vi "Error File Logger.vi"(0 "errlog Name":string="Errors.log", 1 "Module":string, 2 "Clear Error?":bool=TRUE, 3 "ContainerFolder(Empty for Application Folder)":path, 5 "error in (no error)":errorcluster) -> (4 "Error Log":string, 6 "error out":errorcluster)   [LabVIEW 2017]
doc: "Appends the error on the error in cluster to a log file, creating the folder and file when they do not exist, and returns the log text. Wire Clear Error? to clear the error after logging, and ContainerFolder to choose where the log is written (empty uses the application folder)."
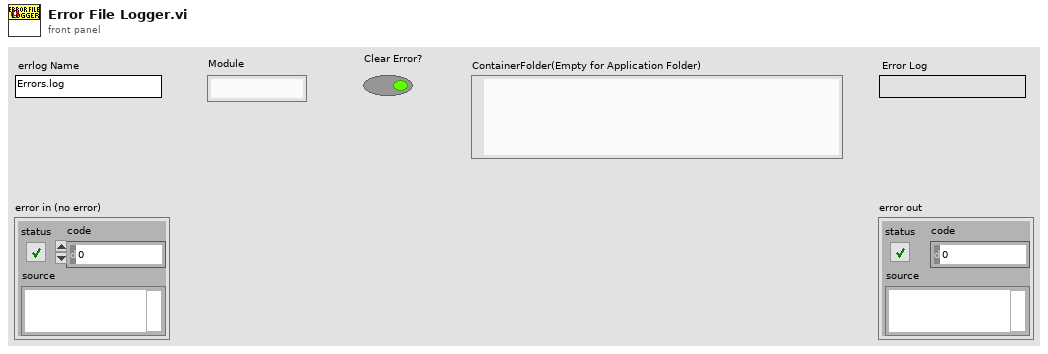
[diagram p1: front panel]
types:
  T1 = enum16{"open", "replace", "create", "open or create", "replace or create", "replace or create with confirmation"}
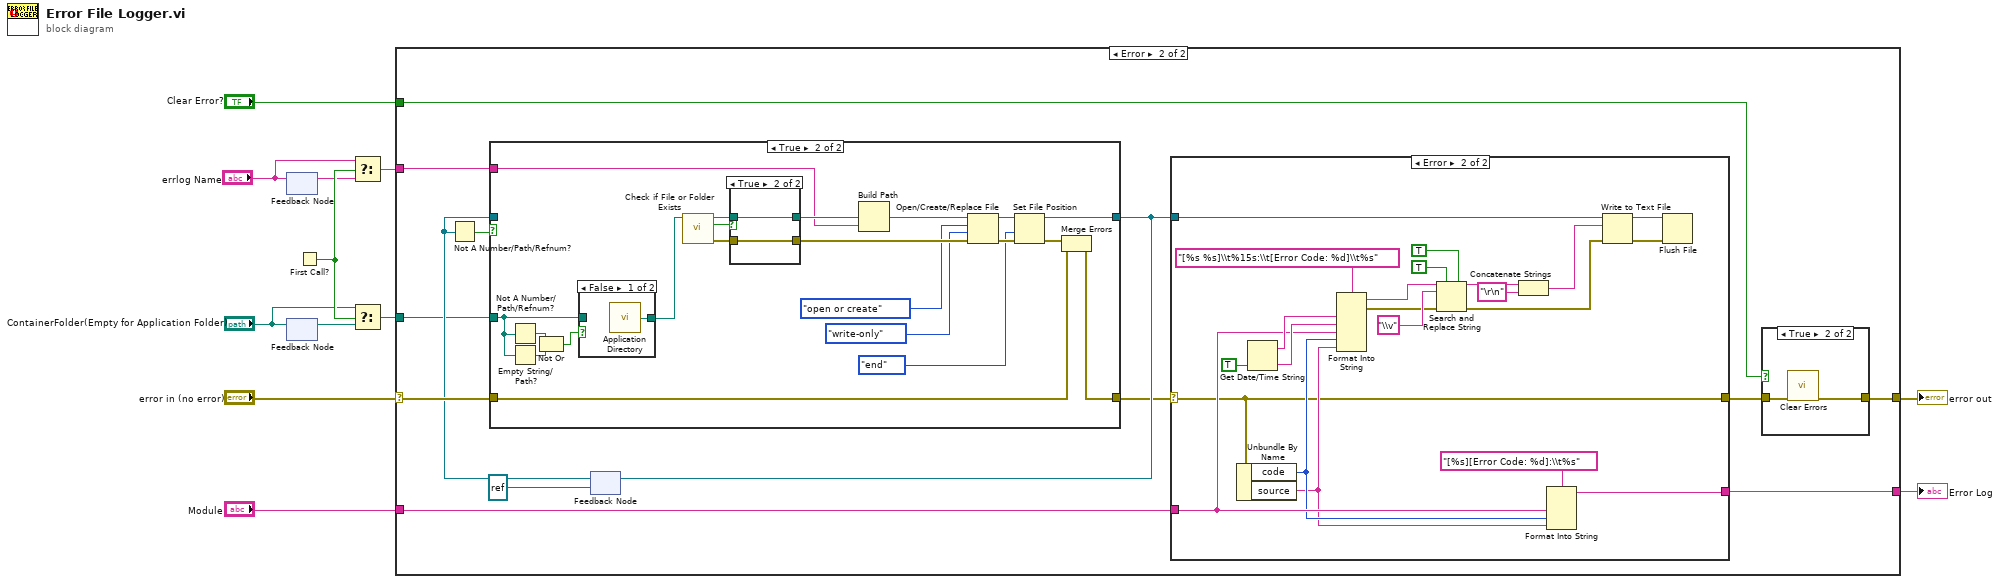
[diagram p0: block diagram]
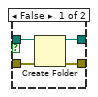
[diagram p7: hidden frame]
diagram:
  n1 = feedback-in #1("errlog Name") -> ()
  n2 = feedback #1() -> (w5:string)  [unwired: 1 in]
  n3 = feedback #2() -> (w6:path)  [unwired: 1 in]
  n4 = feedback-in #2("ContainerFolder(Empty for Application Folder)") -> ()
  n5 = First Call?() -> (First Call?: T/F=w7:bool)
  n6 = Select(t="errlog Name", s=w7, f=w5) -> (s? t:f=w3:string)
  n7 = Select(t="ContainerFolder(Empty for Application Folder)", s=w7, f=w6) -> (s? t:f=w2:path)
  n8 = case shown="Error" "error in (no error)" {
    selector: "error in (no error)" -> [w13 w26]
    tunnel: "Module" -> [_ w20]
    tunnel: [w13 w15] -> w10
    tunnel: w3 -> [_ w22]
    tunnel: [_ w17] -> w9
    tunnel: w2 -> [_ w16]
    tunnel: "Clear Error?" -> [_ w14]
    frame No Error {
    }
    frame Error {
      n9 = feedback #3(refnum<file> refnum ("Error Log File Refnum")) -> (w24:refnum<file>)
      n10 = Not A Number/Path/Refnum?(number/path/refnum=w24) -> (NaN/Path/Refnum?=w25:bool)
      n11 = case shown="True" w25 {
        tunnel: w26 -> [w53 w59]
        tunnel: [w53 w60] -> w19
        tunnel: [w54 w63] -> w21
        tunnel: w24 -> [w54 _]
        tunnel: w22 -> [_ w61]
        tunnel: w16 -> [_ w57]
        frame False {
        }
        frame True {
          n12 = Not A Number/Path/Refnum?(number/path/refnum=w57) -> (NaN/Path/Refnum?=w56:bool)
          n13 = Empty String/Path?(string/path=w57) -> (empty?=w55:bool)
          n14 = Not Or(1:w55, 2:w56) -> (0:w58:bool)
          n15 = case shown="False" w58 {
            tunnel: [w76 w77] -> w70
            tunnel: w57 -> [_ w77]
            frame False {
              n16 = call <vilib>:"Application Directory.vi"() -> ("Application Directory"=w76:path)
            }
            frame True {
            }
          }
          n17 = call <vilib>:"Check if File or Folder Exists.vi"("path"=w70) -> ("error out"=w75:errorcluster, "file or folder exists?"=w71:bool, "dup path"=w73:path)  [unwired: 8 in]
          n18 = case shown="True" w71 {
            tunnel: w75 -> [w81 w82]
            tunnel: [w80 w82] -> w72
            tunnel: w73 -> [w79 w83]
            tunnel: [w78 w83] -> w74
            frame False {
              n19 = Create Folder(path (use dialog)=w79, error in=w81) -> (created path=w78:path, error out=w80:errorcluster)  [unwired: 1 in, 1 out]
            }
            frame True {
            }
          }
          n20 = Build Path(base path=w74, name or relative path=w61) -> (appended path=w67:path)
          n21 = Open/Create/Replace File(file path (use dialog)=w67, error in=w72, operation (0:open)=T1."open or create", access (0:read/write)=enum16{"read/write", "read-only", "write-only"}."write-only") -> (refnum out=w66:refnum<file>, error out=w65:errorcluster)  [unwired: 2 in, 1 out]
          n22 = Set File Position(refnum=w66, from (0:start)=enum16{"start", "end", "current"}."end", error in=w65) -> (refnum out=w63:refnum<file>, error out=w62:errorcluster)  [unwired: 1 in]
          n23 = Merge Errors(w62, w59) -> (w60:errorcluster)
        }
      }
      n24 = feedback-in #3(w21) -> ()
      n25 = case shown="Error" w19 {
        selector: w19 -> [w30 w31]
        tunnel: w21 -> [_ w38]
        tunnel: w20 -> [_ w35]
        tunnel: [_ w32] -> w17
        tunnel: [w30 w31] -> w18
        frame No Error {
        }
        frame Error {
          n26 = Unbundle By Name(w31) -> ("code"=w34:i32, "source"=w33:string)
          n27 = Get Date/Time String(want seconds? (F)=TRUE) -> (date string=w50:string, time string=w49:string)  [unwired: 2 in]
          n28 = Format Into String(format string="[%s %s]\\t%15s:\\t[Error Code: %d]\\t%s", w50, w49, w35, w34, w33) -> (resulting string=w45:string, error out=w43:errorcluster)  [unwired: 2 in]
          n29 = Search and Replace String(replace all?=TRUE ("replace all? (F)"), multiline?=TRUE ("ignore case? (F)"), input string=w45, search string="\\v" ("string"), error in=w43) -> (result string=w37:string, error out=w39:errorcluster)  [unwired: 3 in, 2 out]
          n30 = Concatenate Strings(w37, "\r\n" ("string")) -> (w47:string)
          n31 = Format Into String(format string="[%s][Error Code: %d]:\\t%s", w35, w34, w33) -> (resulting string=w32:string)  [unwired: 2 in, 1 out]
          n32 = Write to Text File(file (use dialog)=w38, text=w47, error in=w39) -> (refnum out=w40:refnum<file>, error out=w48:errorcluster)  [unwired: 1 in, 1 out]
          n33 = Flush File(refnum=w40, error in=w48) -> ()  [unwired: 2 out]
        }
      }
      n34 = case shown="True" w14 {
        tunnel: w18 -> [w27 w29]
        tunnel: [w27 w28] -> w15
        frame False {
        }
        frame True {
          n35 = call <vilib>:"Clear Errors.vi"("error in (no error)"=w29) -> ("error out"=w28:errorcluster)  [unwired: 5 in, 1 out]
        }
      }
    }
  }
  "error out" <- w10
  "Error Log" <- w9
